vi "GFITS_execPostImg.vi"(8 "error in":errorcluster, 10 "image name":string, 11 "Database RefNum in":T1) -> (0 "error out":errorcluster)   [LabVIEW 2016]
uses:
  DBSHAND/private/vis/DatabaseHand_RefNum.ctl
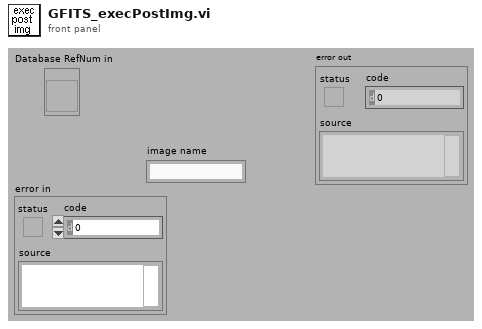
[diagram p1: front panel]
types:
  T1 = typedef "DatabaseHand_RefNum.ctl" = refnum<vi>
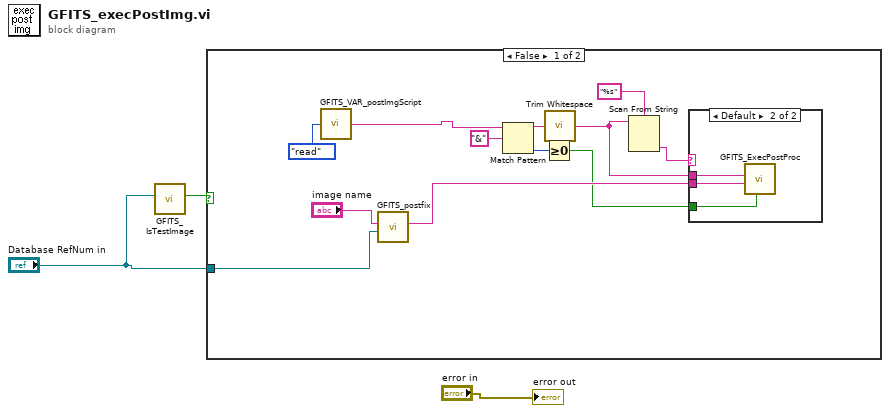
[diagram p0: block diagram]
diagram:
  n1 = call "GFITS_IsTestImage.vi"("Database RefNum in"="Database RefNum in") -> ("testonly"=w2:bool)  [unwired: 10 out]
  n2 = case shown="False" w2 {
    tunnel: "Database RefNum in" -> [w4 _]
    frame False {
      n3 = call "GFITS_VAR_postImgScript.vi"("action"=enum16{"read", "write"}."read") -> ("script name out"=w9:string)  [unwired: 1 in, 13 out]
      n4 = call "GFITS_postfix.vi"("Database RefNum in"=w4, "imname in"="image name") -> ("imname out"=w13:string)  [unwired: 9 out]
      n5 = Match Pattern(string=w9, regular expression="&") -> (before substring=w10:string, offset past match=w11:i32)  [unwired: 3 out]
      n6 = Greater Or Equal To 0?(x=w11) -> (x >= 0?=w8:bool)
      n7 = call <vilib>:"Trim Whitespace.vi"("string"=w10) -> ("trimmed string"=w6:string)  [unwired: 1 in]
      n8 = Scan From String(format string="%s", input string=w6) -> (output 1=w7:string)  [unwired: 2 in, 4 out]
      n9 = case shown="Default" w7 {
        tunnel: w13 -> [_ w18]
        tunnel: w6 -> [_ w17]
        tunnel: w8 -> [_ w16]
        frame "", "false", "no", "none", "off" {
        }
        frame Default {
          n10 = call "GFITS_ExecPostProc.vi"("background"=w16, "impath"=w18, "postproc"=w17) -> ()  [unwired: 2 in, 7 out]
        }
      }
    }
    frame True {
    }
  }
  "error out" <- "error in"
